vi "iRobot UART Read Simple Packet.vi"(8 "error in":errorcluster, 9 "timeout (ms) (-1)":i32=-1, 10 "packet configuration":T2, 11 "UART session":T1) -> (0 "error out":errorcluster, 1 "timed out?":bool, 2 "payload":u8[](array[numeric]), 3 "UART session":T1, 4 "cx fail":i32, 5 "bytes discarded":i32, 6 "cx pass":i32)   [LabVIEW 2013]
doc: "Read a simple VISA packet of the form [header] [payload size] [payload] [(optional) checksum]\n\nThis VI blocks until a packet is received, or until a timeout occurs."
uses:
  iRobot UART Simple Packet Configuration.ctl
  iRobot UART Port Type.ctl
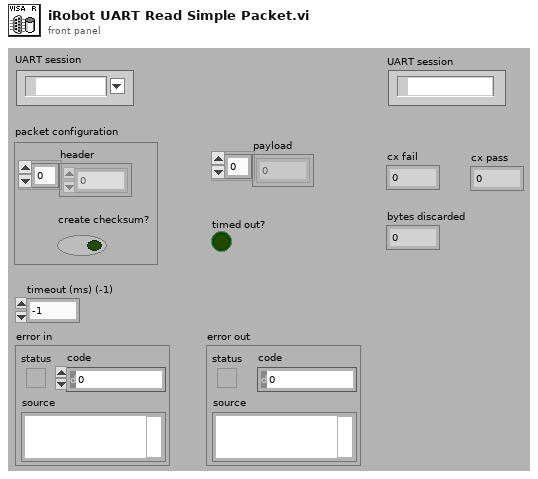
[diagram p1: front panel]
types:
  T1 = typedef "iRobot UART Port Type.ctl" = refnum<visa-resource-name>
  T2 = typedef "iRobot UART Simple Packet Configuration.ctl" = cluster{"header":u8[], "create checksum?":bool}
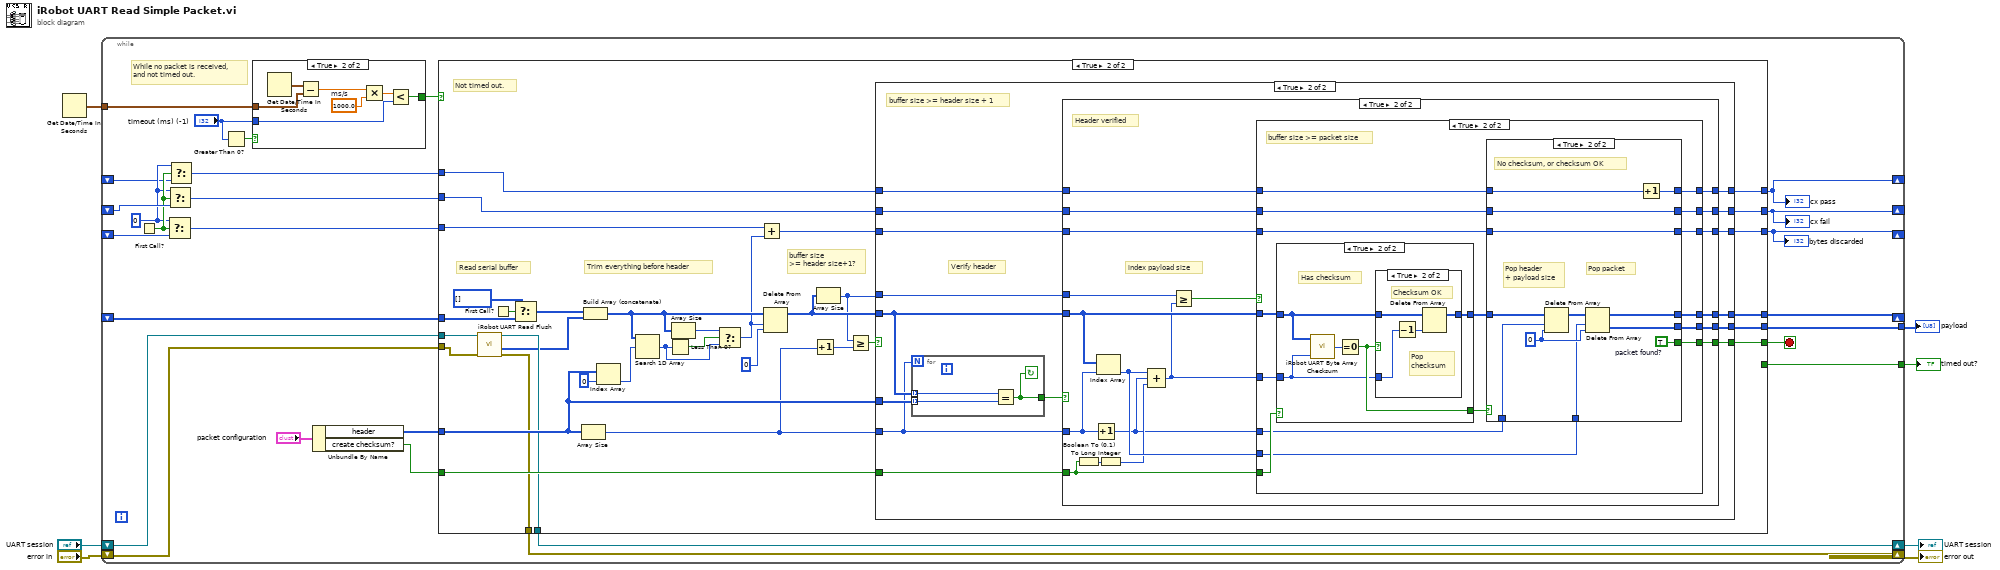
[diagram p0: block diagram]
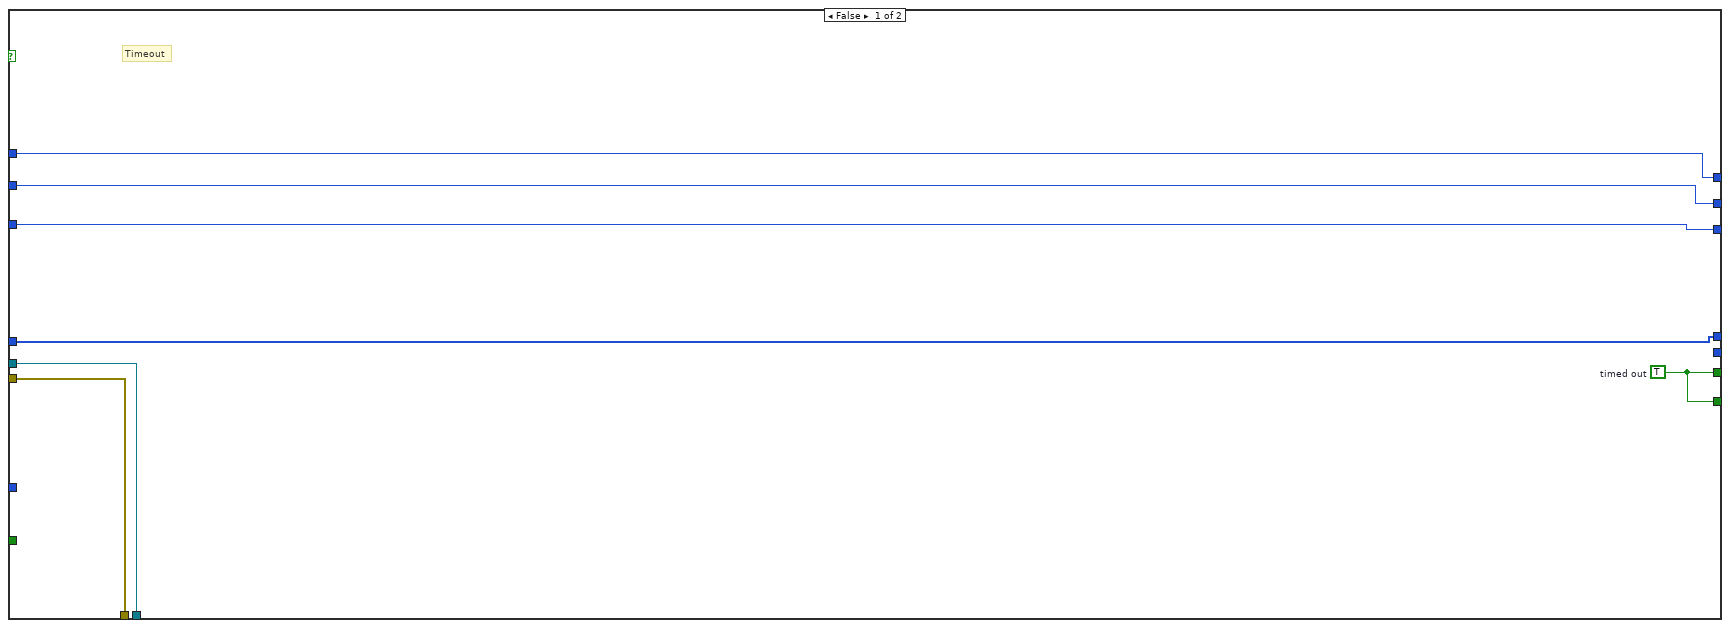
[diagram p2: hidden frame]
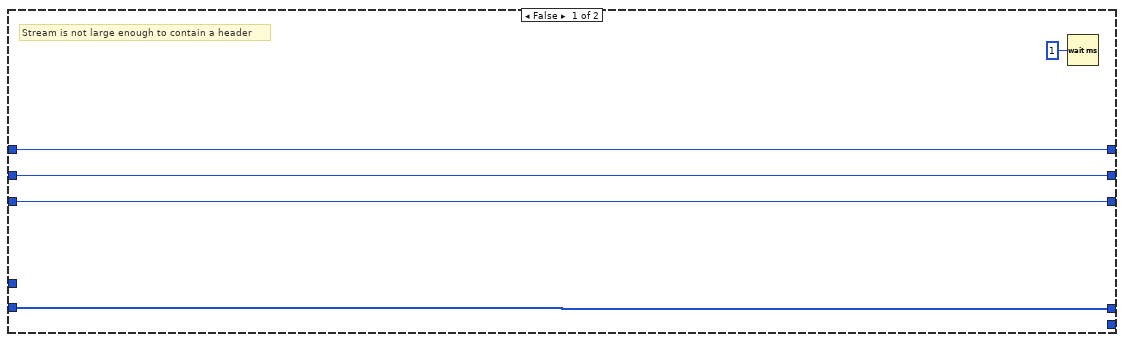
[diagram p3: hidden frame]
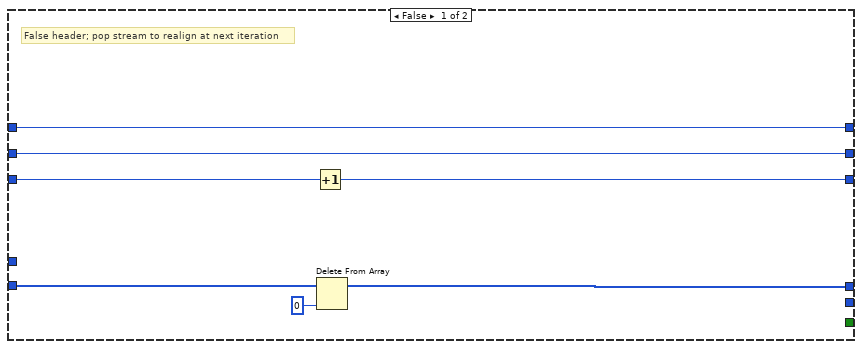
[diagram p4: hidden frame]
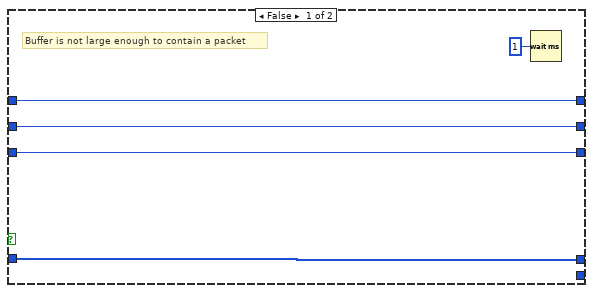
[diagram p5: hidden frame]
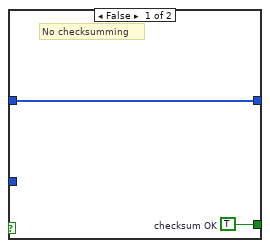
[diagram p6: hidden frame]
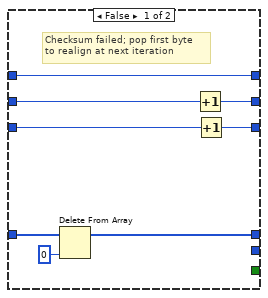
[diagram p8: hidden frame]
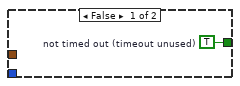
[diagram p9: hidden frame]
diagram:
  n1 = Get Date/Time In Seconds() -> (seconds since 1Jan1904=w6:timestamp)
  n2 = while {
    shift-right: [w15] -> _
    shift-left: _ -> [w33]
    tunnel: [w34] -> w7
    tunnel: w6 -> [w31]
    shift-right: [w24] -> w1
    shift-left: "UART session" -> [w18]
    shift-right: [w23] -> w5
    shift-left: "error in" -> [w22]
    tunnel: [w21] -> w3
    shift-right: [w13] -> _
    shift-left: _ -> [w20]
    shift-right: [w14] -> _
    shift-left: _ -> [w17]
    shift-right: [w8] -> _
    shift-left: _ -> [w10]
    stop <- w32 stop-if-true
    w11 = 0 ("bytes discarded")
    # "While no packet is received,\nand not timed out."
    n3 = First Call?() -> (First Call?: T/F=w12:bool)
    n4 = Select(t=w11, s=w12, f=w20) -> (s? t:f=w19:i32)
    n5 = Select(t=w11, s=w12, f=w17) -> (s? t:f=w16:i32)
    n6 = Select(t=w11, s=w12, f=w10) -> (s? t:f=w9:i32)
    n7 = Greater Than 0?(x="timeout (ms) (-1)") -> (x > 0?=w30:bool)
    n8 = case shown="True" w30 {
      tunnel: w31 -> [_ w184]
      tunnel: "timeout (ms) (-1)" -> [_ w180]
      tunnel: [w178 w179] -> w28
      frame False {
        w178 = TRUE  # not timed out (timeout unused)
      }
      frame True {
        w182 = 1000.0  # ms/s
        n9 = Get Date/Time In Seconds() -> (seconds since 1Jan1904=w185:timestamp)
        n10 = Subtract(x=w185, y=w184) -> (x-y=w183:dbl)
        n11 = Multiply(x=w183, y=w182) -> (x*y=w181:dbl)
        n12 = Less?(x=w181, y=w180) -> (x < y?=w179:bool)
      }
    }
    n13 = Unbundle By Name("packet configuration") -> ("header"=w26:u8[], "create checksum?"=w25:bool)
    n14 = case shown="True" w28 {
      tunnel: [w39 w46] -> w23
      tunnel: [w41 w75] -> w15
      tunnel: [w40 w47] -> w24
      tunnel: w26 -> [_ w74]
      tunnel: w25 -> [_ w73]
      tunnel: [_ w72] -> w34
      tunnel: w33 -> [w41 w71]
      tunnel: w18 -> [w40 w49]
      tunnel: w22 -> [w39 w48]
      tunnel: [w38 w70] -> w32
      tunnel: [w38 _] -> w21
      tunnel: w19 -> [w36 w69]
      tunnel: [w36 w68] -> w13
      tunnel: [w37 w67] -> w14
      tunnel: w16 -> [w37 w66]
      tunnel: w9 -> [w35 w43]
      tunnel: [w35 w42] -> w8
      frame False {
        w38 = TRUE  # timed out
        # "Timeout"
      }
      frame True {
        # "buffer size\n>= header size+1?"
        # "Trim everything before header"
        # "Read serial buffer"
        # "Not timed out."
        n15 = call "iRobot UART Read Flush.vi"("error in"=w48, "UART port in"=w49) -> ("error out"=w46:errorcluster, "data"=w45:u8[], "UART port out"=w47:T1)  [unwired: 7 in]
        n16 = First Call?() -> (First Call?: T/F=w51:bool)
        n17 = Select(t=u8[] [] ("payload elements"), s=w51, f=w71) -> (s? t:f=w50:u8[])
        n18 = Array Size(array=w74) -> (size(s)=w56:i32)
        n19 = Build Array (concatenate)(w50, w45) -> (w65:u8[])
        n20 = Index Array(array=w74, index=0) -> (element=w58:u8)
        n21 = Search 1D Array(1D array=w65, element=w58) -> (index of element=w60:i32)  [unwired: 1 in]
        n22 = Less Than 0?(x=w60) -> (x < 0?=w61:bool)
        n23 = Array Size(array=w65) -> (size(s)=w63:i32)
        n24 = Select(t=w63, s=w61, f=w60) -> (s? t:f=w53:i32)
        n25 = Add(x=w69, y=w53) -> (x+y=w52:i32)
        n26 = Delete From Array(array=w65, length=w53, index=0 ("t")) -> (array with subset deleted=w57:u8[])  [unwired: 1 out]
        n27 = Increment(x=w56) -> (x+1=w54:i32)
        n28 = Array Size(array=w57) -> (size(s)=w55:i32)
        n29 = Greater Or Equal?(x=w55, y=w54) -> (x >= y?=w64:bool)
        n30 = case shown="True" w64 {
          tunnel: [w80 w93] -> w75
          tunnel: w57 -> [w80 w94]
          tunnel: w74 -> [_ w92]
          tunnel: w56 -> [_ w83]
          tunnel: w73 -> [_ w91]
          tunnel: w55 -> [_ w90]
          tunnel: [_ w89] -> w72
          tunnel: [_ w88] -> w70
          tunnel: w52 -> [w79 w87]
          tunnel: [w79 w86] -> w68
          tunnel: [w78 w85] -> w67
          tunnel: w66 -> [w78 w84]
          tunnel: w43 -> [w77 w82]
          tunnel: [w77 w81] -> w42
          frame False {
            # "Stream is not large enough to contain a header"
            n31 = Wait (ms)(milliseconds to wait=u32 1) -> ()  [unwired: 1 out]
          }
          frame True {
            # "Verify header"
            # "buffer size >= header size + 1"
            n32 = for {
              N: w83 -> [_]
              tunnel: w92 -> [w176] mode=indexing
              tunnel: [w177] -> w95
              tunnel: w94 -> [w175] mode=indexing
              stop <- w177 continue-if-true
              n33 = Equal?(x=w175, y=w176) -> (x = y?=w177:bool)
            }
            n34 = case shown="True" w95 {
              tunnel: [w100 w121] -> w93
              tunnel: w94 -> [w101 w120]
              tunnel: w83 -> [_ w106]
              tunnel: w91 -> [_ w118]
              tunnel: w90 -> [_ w119]
              tunnel: [_ w112] -> w89
              tunnel: [_ w111] -> w88
              tunnel: w87 -> [w99 w110]
              tunnel: [w98 w109] -> w86
              tunnel: [w97 w108] -> w85
              tunnel: w84 -> [w97 w107]
              tunnel: w82 -> [w96 w104]
              tunnel: [w96 w103] -> w81
              frame False {
                # "False header; pop stream to realign at next iteration"
                n35 = Increment(x=w99) -> (x+1=w98:i32)
                n36 = Delete From Array(array=w101, index=0) -> (array with subset deleted=w100:u8[])  [unwired: 1 in, 1 out]
              }
              frame True {
                # "index payload size"
                # "Header verified"
                n37 = Boolean To (0,1)(Boolean=w118) -> (0, 1=w117:i16)
                n38 = Increment(x=w106) -> (x+1=w105:i32)
                n39 = Index Array(array=w120, index=w106) -> (element=w115:u8)
                n40 = To Long Integer(number=w117) -> (32bit integer=w113:i32)
                n41 = Compound Arithmetic op=ADD(w115, w105, w113) -> (w114:i32)
                n42 = Greater Or Equal?(x=w119, y=w114) -> (x >= y?=w116:bool)
                n43 = case shown="True" w116 {
                  tunnel: [w126 w142] -> w121
                  tunnel: w120 -> [w126 w139]
                  tunnel: w118 -> [_ w138]
                  tunnel: w105 -> [_ w136]
                  tunnel: w115 -> [_ w135]
                  tunnel: w114 -> [_ w137]
                  tunnel: [_ w134] -> w112
                  tunnel: [_ w133] -> w111
                  tunnel: w110 -> [w125 w131]
                  tunnel: [w125 w132] -> w109
                  tunnel: [w124 w129] -> w108
                  tunnel: w107 -> [w124 w130]
                  tunnel: w104 -> [w123 w128]
                  tunnel: [w123 w127] -> w103
                  frame False {
                    # "Buffer is not large enough to contain a packet"
                    n44 = Wait (ms)(milliseconds to wait=u32 1) -> ()  [unwired: 1 out]
                  }
                  frame True {
                    # "buffer size >= packet size"
                    n45 = case shown="True" w138 {
                      tunnel: w139 -> [w144 w148]
                      tunnel: [w143 w146] -> w141
                      tunnel: [w144 w147] -> w140
                      tunnel: w137 -> [_ w145]
                      frame False {
                        w143 = TRUE  # checksum OK
                        # "No checksumming"
                      }
                      frame True {
                        # "Has checksum"
                        n46 = call "iRobot UART Byte Array Checksum.vi"("Number of Values (-1)"=w145, "Byte Array"=w148) -> ("Checksum"=w149:u8)  [unwired: 1 in]
                        n47 = Equal To 0?(x=w149) -> (x = 0?=w146:bool)
                        n48 = case shown="True" w146 {
                          tunnel: w148 -> [w150 w154]
                          tunnel: [w150 w153] -> w147
                          tunnel: w145 -> [_ w152]
                          frame False {
                            # "Checksum FAIL"
                          }
                          frame True {
                            # "Pop\nchecksum"
                            # "Checksum OK"
                            n49 = Decrement(x=w152) -> (x-1=w151:i32)
                            n50 = Delete From Array(array=w154, index=w151) -> (array with subset deleted=w153:u8[])  [unwired: 1 in, 1 out]
                          }
                        }
                      }
                    }
                    n51 = case shown="True" w141 {
                      tunnel: [w160 w174] -> w142
                      tunnel: w140 -> [w161 w173]
                      tunnel: w136 -> [_ w165]
                      tunnel: w135 -> [_ w170]
                      tunnel: [_ w169] -> w134
                      tunnel: [_ w168] -> w133
                      tunnel: [w158 w167] -> w132
                      tunnel: w131 -> [w159 w167]
                      tunnel: w130 -> [w157 w166]
                      tunnel: [w156 w166] -> w129
                      tunnel: [w155 w163] -> w127
                      tunnel: w128 -> [w155 w164]
                      frame False {
                        # "Checksum failed; pop first byte\nto realign at next iteration"
                        n52 = Delete From Array(array=w161, index=0) -> (array with subset deleted=w160:u8[])  [unwired: 1 in, 1 out]
                        n53 = Increment(x=w157) -> (x+1=w156:i32)
                        n54 = Increment(x=w159) -> (x+1=w158:i32)
                      }
                      frame True {
                        w168 = TRUE  # packet found?
                        w171 = 0 ("index")
                        # "Pop header\n+ payload size"
                        # "Pop packet"
                        # "No checksum, or checksum OK"
                        n55 = Delete From Array(array=w173, length=w165, index=w171) -> (array with subset deleted=w172:u8[])  [unwired: 1 out]
                        n56 = Delete From Array(array=w172, length=w170, index=w171) -> (deleted portion=w169:u8[], array with subset deleted=w174:u8[])
                        n57 = Increment(x=w164) -> (x+1=w163:i32)
                      }
                    }
                  }
                }
              }
            }
          }
        }
      }
    }
    "cx fail" <- w14
    "bytes discarded" <- w13
    "cx pass" <- w8
  }
  "error out" <- w5
  "payload" <- w7
  "timed out?" <- w3
  "UART session" <- w1
